vi "OPERATEUR.vi"(8 "errin":errorcluster, 11 "IN":string) -> (0 "error out":errorcluster caption="errout", 3 "Dataout":string)   [LabVIEW 2020]
uses:
  <userlib>/Alex.vi/FGV.ctl
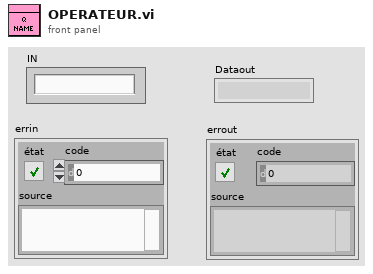
[diagram p1: front panel]
types:
  T1 = typedef "FGV.ctl" = enum16{"GET", "SET", "RAZ"}
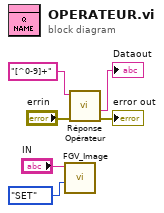
[diagram p0: block diagram]
diagram:
  n1 = call <userlib>:"FGV_Image.vi"("Énum"=FGV."SET", "IN"="IN") -> ()  [unwired: 8 in, 2 out]
  n2 = call "Réponse Opérateur.vi"("errin"="errin", "expression régulière"="[^0-9]+") -> ("errout"=→"error out":errorcluster, "toute l'expression"=→"Dataout":string)  [unwired: 6 in, 2 out]
